vi "Positioner.vi"(8 "error in":errorcluster) -> (0 "error out":errorcluster)   [LabVIEW 2022 SP3]
uses:
  Global 2.vi
  Global 1.vi
  Newport.XPS.CommandInterface
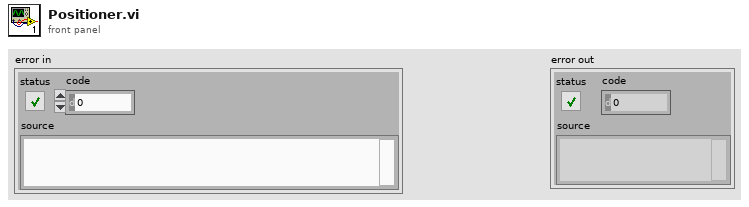
[diagram p1: front panel]
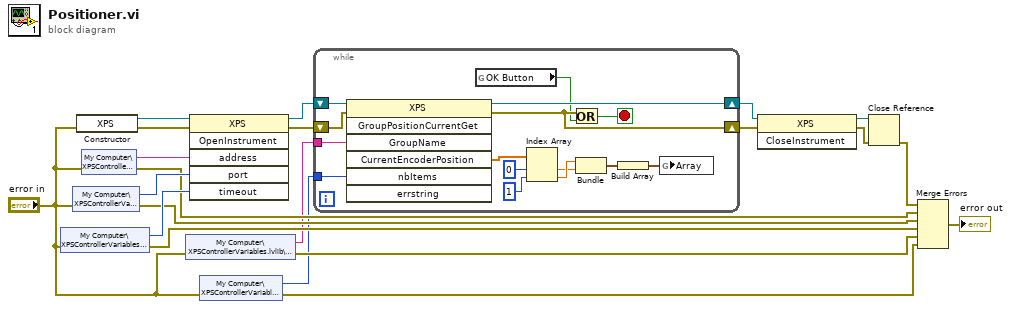
[diagram p0: block diagram]
diagram:
  n1 = shared-variable "My Computer\\XPSControllerVariables.lvlib\\Timeout"(error in="error in") -> (w17:i16, error out=w12:errorcluster)
  n2 = shared-variable "My Computer\\XPSControllerVariables.lvlib\\Port"(error in="error in") -> (w18:i16, error out=w13:errorcluster)
  n3 = constructor class="XPS"(error in="error in") -> (reference out=w21:refnum<k24>, error out=w20:errorcluster)  [unwired: 2 in, 1 out]
  n4 = shared-variable "My Computer\\XPSControllerVariables.lvlib\\IP"(error in="error in") -> (w19:string, error out=w14:errorcluster)
  n5 = shared-variable "My Computer\\XPSControllerVariables.lvlib\\GroupName"(error in="error in") -> (w5:string, error out=w11:errorcluster)
  n6 = invoke class="XPS" method="OpenInstrument"(reference=w21, error in=w20, "address"=w19, "port"=w18, "timeout"=w17) -> (reference out=w9:refnum<k24>, error out=w8:errorcluster)  [unwired: 1 in, 4 out]
  n7 = shared-variable "My Computer\\XPSControllerVariables.lvlib\\nbitem"(error in="error in") -> (w4:i16, error out=w2:errorcluster)
  n8 = while {
    tunnel: w5 -> [w33]
    tunnel: w4 -> [w32]
    shift-right: [w34] -> w7
    shift-left: w9 -> [w36]
    shift-right: [w31] -> w6
    shift-left: w8 -> [w35]
    stop <- w30 stop-if-true
    n9 = invoke class="XPS" method="GroupPositionCurrentGet"(reference=w36, error in=w35, "GroupName"=w33, "nbItems"=w32) -> (reference out=w34:refnum<k24>, error out=w31:errorcluster, "CurrentEncoderPosition"=w29:dbl[])  [unwired: 3 in, 4 out]
    n10 = global read "Global 2.vi" "OK Button"() -> (w24:bool)
    n11 = Index Array(array=w29, index #1=0, index #2=1) -> (element #1=w22:dbl, element #2=w23:dbl)
    n12 = Or(x=w31, y=w24) -> (x .or. y?=w30:bool)
    n13 = Bundle(w23, w22) -> (w26:cluster{dbl, dbl})  [unwired: 1 in]
    n14 = Build Array(w26) -> (w25:cluster{dbl, dbl}[])
    n15 = global write "Global 1.vi" "Array"(w25) -> ()
  }
  n16 = invoke class="XPS" method="CloseInstrument"(reference=w7, error in=w6) -> (reference out=w16:refnum<k24>, error out=w15:errorcluster)  [unwired: 1 in, 1 out]
  n17 = Close Reference(reference=w16, error in (no error)=w15) -> (error out=w10:errorcluster)
  n18 = Merge Errors(w10, w14, w13, w12, w11, w2) -> (→"error out":errorcluster)
